vi "Calculate Default Splitter Positions.vi"(8 "error in":errorcluster, 11 "Manual UI in":refnum<class "Manual UI.lvclass">) -> (0 "error out":errorcluster, 3 "Manual UI out":refnum<class "Manual UI.lvclass">)   [LabVIEW 2023, in "Manual UI.lvlib" / "Manual UI.lvclass"]
uses:
  Project/Manual UI.lvclass
  C:/Users/Public/Documents/Development/builds/Engine/Engine.lvlibp/Project/Engine.lvclass
  Project/Manual UI.lvclass/Manual UI.ctl
  builds/Engine/Engine.lvlibp/Accessors/Read VI_Ref.vi
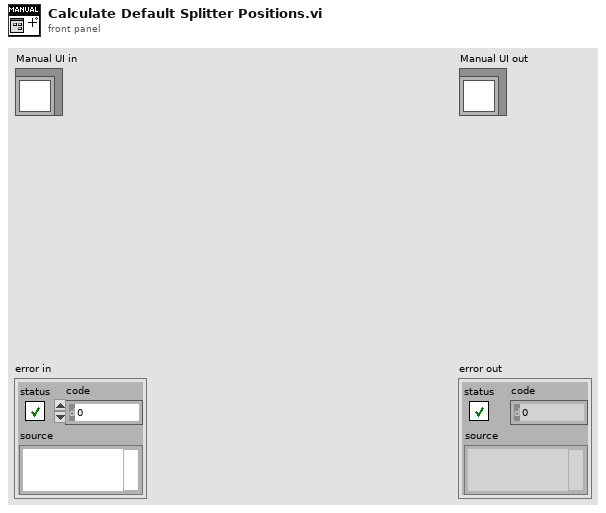
[diagram p1: front panel]
types:
  T1 = typedef "LVRectTypeDef.ctl" = cluster{"Left":i16, "Top":i16, "Right":i16, "Bottom":i16}
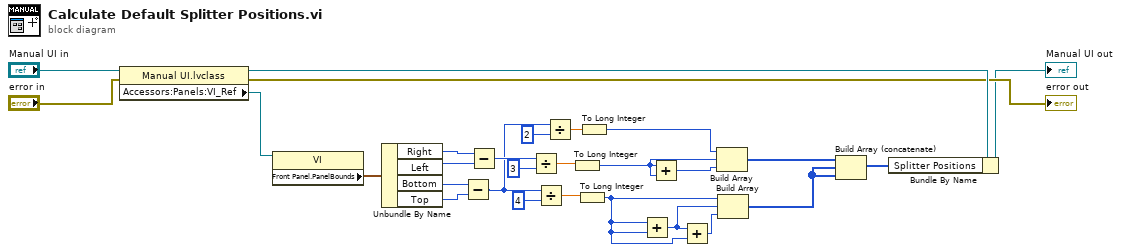
[diagram p0: block diagram]
diagram:
  n1 = property class="Manual UI.lvclass"(reference="Manual UI in", error in="error in") -> (reference out=w26:refnum<class "Manual UI.lvclass">, error out=→"error out":errorcluster, "Accessors:Panels:VI_Ref"=w24:refnum<vi>)
  n2 = property class="VI"(reference=w24) -> ("Front Panel.PanelBounds"=w23:T1)  [unwired: 1 in, 2 out]
  n3 = Unbundle By Name(w23) -> ("Right"=w22:i16, "Left"=w21:i16, "Bottom"=w19:i16, "Top"=w20:i16)
  n4 = Subtract(x=w19, y=w20) -> (x-y=w4:i16)
  n5 = Subtract(x=w22, y=w21) -> (x-y=w18:i16)
  n6 = Divide(x=w18, y=i16 3) -> (x/y=w16:dbl)
  n7 = Divide(x=w4, y=i16 4) -> (x/y=w15:dbl)
  n8 = Divide(x=w4, y=i16 2) -> (x/y=w2:dbl)
  n9 = To Long Integer(number=w16) -> (32bit integer=w12:i32)
  n10 = To Long Integer(number=w15) -> (32bit integer=w6:i32)
  n11 = To Long Integer(number=w2) -> (32bit integer=w1:i32)
  n12 = Add(x=w6, y=w6) -> (x+y=w8:i32)
  n13 = Add(x=w12, y=w12) -> (x+y=w13:i32)
  n14 = Add(x=w8, y=w6) -> (x+y=w7:i32)
  n15 = Build Array(w1, w12, w13) -> (w11:i32[])
  n16 = Build Array(w6, w8, w7) -> (w5:i32[])
  n17 = Build Array (concatenate)(w11, w5, w5) -> (w9:i32[])
  n18 = Bundle By Name(cluster=w26, "Splitter Positions"=w9) -> (→"Manual UI out":refnum<class "Manual UI.lvclass">)
